vi "COTP - Build Connection Request Packet.vi"(8 "error in (no error)":errorcluster, 11 "S7NetCom in":refnum<class "S7NetCom.lvclass">) -> (0 "error out":errorcluster, 2 "COTP Connection Request":T1 format="0x%02x", 3 "S7NetCom out":refnum<class "S7NetCom.lvclass">)   [LabVIEW 2014, in "S7NetCom.lvclass"]
doc: "____\nCopyright (c) 2019 Hampel Software Engineering (HSE), released under BSD license. More info can be found on https://dokuwiki.hampel-soft.com/code/hse/s7netcom. Original code published by Marc Christenson, Sisu Devices."
uses:
  S7NetCom.lvclass
  Controls/S7NetCom_HexByteArray.ctl
  Controls/S7NetCom_HexByte.ctl
  S7NetCom.lvclass/S7NetCom.ctl
  Accessors/Get Slot Number.vi
  Accessors/Get Rack Number.vi
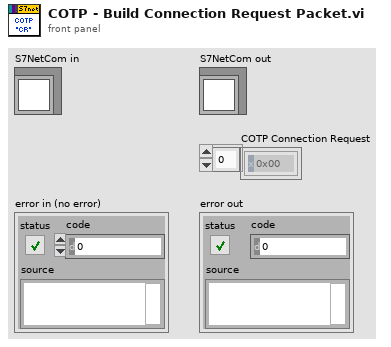
[diagram p1: front panel]
types:
  T1 = typedef "S7NetCom.lvclass/S7NetCom_HexByteArray.ctl" = T2[]
  T2 = typedef "S7NetCom.lvclass/S7NetCom_HexByte.ctl" = u8
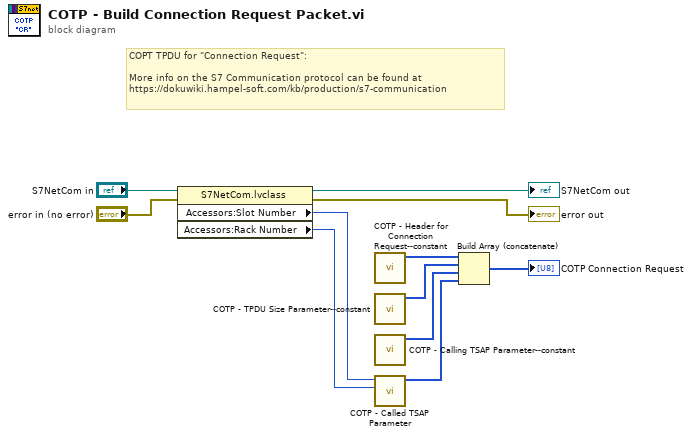
[diagram p0: block diagram]
diagram:
  # "COPT TPDU for \"Connection Request\":\n\nMore info on the S7 Communication protocol can be found at\nhttps://dokuwiki.hampel-soft.com/kb/production/s7-communication"
  n1 = property class="S7NetCom.lvclass"(reference="S7NetCom in", error in="error in (no error)") -> (reference out=→"S7NetCom out":refnum<class "S7NetCom.lvclass">, error out=→"error out":errorcluster, "Accessors:Slot Number"=w2:u8, "Accessors:Rack Number"=w1:u8)
  n2 = call "COTP - Header for Connection Request--constant.vi"() -> ("COTP CR Header"=w7:T1)  [unwired: 10 in, 1 out]
  n3 = call "COTP - TPDU Size Parameter--constant.vi"() -> ("COTP TPDU Size"=w5:T1)  [unwired: 11 in]
  n4 = call "COTP - Calling TSAP Parameter--constant.vi"() -> ("COTP Calling TSAP"=w4:T1)  [unwired: 11 in]
  n5 = call "COTP - Called TSAP Parameter.vi"("Rack No."=w1, "Slot No."=w2) -> ("COTP Called TSAP"=w3:T1)  [unwired: 9 in]
  n6 = Build Array (concatenate)(w7, w5, w4, w3) -> (→"COTP Connection Request":T1)
